vi "testAssertionFailureMessage.vi"() -> ()   [LabVIEW 2017, in "Assertion.Tests.lvlib" / "AssertNoError.lvlib"]
uses:
  AssertNoError.lvlib
  <vilib>/Utility/error.llb/Error Cluster From Error Code.vi
  <vilib>/ErrorRing/Error Ring.xnode
  Assertion/Assertion.lvlib
panel:
  out "error out":errorcluster
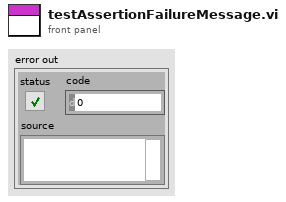
[diagram p1: front panel]
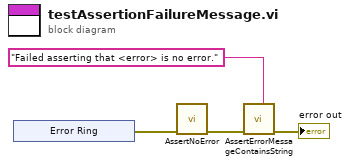
[diagram p0: block diagram]
diagram:
  n1 = xnode "Error Ring"() -> ("error out"=w4:errorcluster)
  n2 = call "AssertNoError.vi"("error in (no error)"=w4) -> ("error out"=w3:errorcluster)  [unwired: 10 in]
  n3 = call "AssertErrorMessageContainsString.vi"("Expected"="Failed asserting that <error> is no error." ("Needle"), "error in (no error)"=w3) -> ("error out"=→"error out":errorcluster)  [unwired: 9 in]
